vi "KMAX test.vi"() -> ()   [LabVIEW 2023]
uses:
  <vilib>/userDefined/High Color/IMAQdx.ctl
panel:
  out "Integration Time Output (ms)":dbl
  in  "IntegrationTime (ms)":dbl=5.0 min=5.0 max=1000.0 step=1.0
  out "error out":errorcluster
  out "XY Graph":T1(graph)
  in  "error in (no error)":errorcluster
  in  "Refnum in":T2
  in  "stop":bool
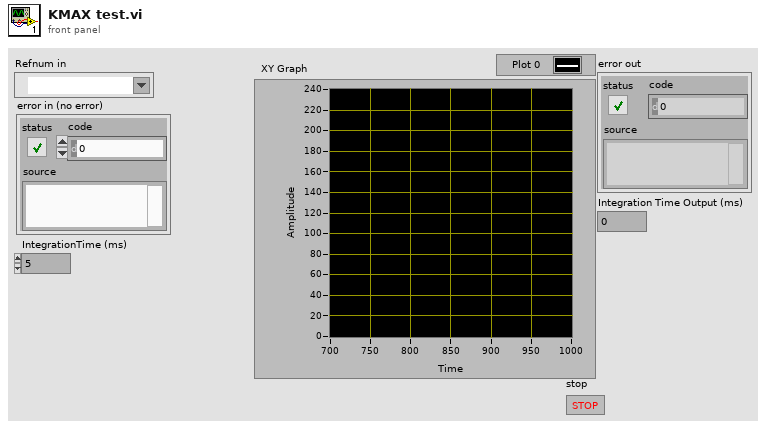
[diagram p1: front panel]
types:
  T1 = cluster{"Wavelengths (nm)":dbl[], "Intensity":sgl[]}
  T2 = typedef "IMAQdx.ctl" = refnum<k21>
  T3 = typedef "IMAQ Image.ctl" = refnum<image>
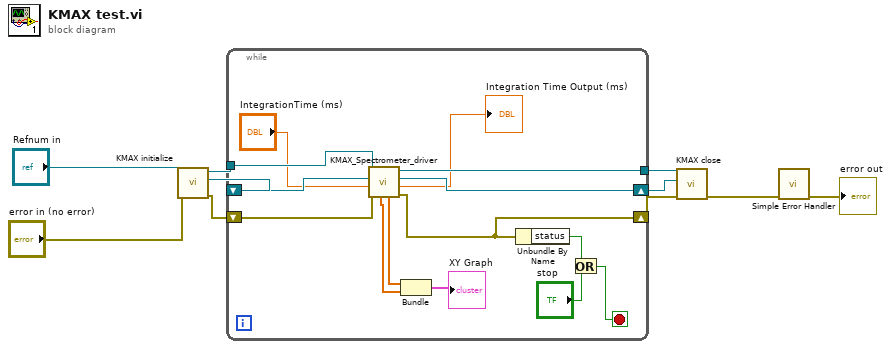
[diagram p0: block diagram]
diagram:
  n1 = call "KMAX initialize.vi"("error in (no error)"="error in (no error)", "Refnum in"="Refnum in") -> ("error out"=w8:errorcluster, "New Image"=w9:T3, "Refnum out"=w1:T2)  [unwired: 7 in]
  n2 = while {
    shift-right: [w24] -> w6
    shift-left: w9 -> [w23]
    shift-right: [w15] -> w5
    shift-left: w8 -> [w22]
    tunnel: w1 -> [w14]
    tunnel: [w13] -> w2
    stop <- w19 stop-if-true
    n3 = call "KMAX_Spectrometer_driver.vi"("error in"=w22, "IntegrationTime (ms)"="IntegrationTime (ms)", "New Image"=w23, "Camera Name"=w14) -> ("error out"=w15:errorcluster, "Integration Time Output (ms)"=→"Integration Time Output (ms)":dbl, "Image Out"=w24:T3, "Session Out"=w13:T2, "Wavelengths (nm)"=w18:dbl[], "Intensity"=w17:sgl[])  [unwired: 2 in]
    n4 = Bundle("Wavelengths (nm)"=w18, "Intensity"=w17) -> (→"XY Graph":T1)  [unwired: 1 in]
    n5 = Unbundle By Name(w15) -> ("status"=w21:bool)
    n6 = Or(x=w21, y="stop") -> (x .or. y?=w19:bool)
  }
  n7 = call "KMAX close.vi"("error in (no error)"=w5, "Image Out"=w6, "Refnum in"=w2) -> ("error out"=w7:errorcluster)  [unwired: 8 in]
  n8 = call <vilib>:"Simple Error Handler.vi"("error in (no error)"=w7) -> ("error out"=→"error out":errorcluster)  [unwired: 1 in, 7 out]
